vi "sortData.vi"(8 "error in (no error)":errorcluster, 9 "data":T1(array[cluster])=[[{"time"=0.0, "Channel"=refnum, "data"=0.8}, {"time"=29.998, "Channel"=refnum, "data"=0.0}], [{"time"=0.0, "Channel"=refnum, "data"=0.74}, {"time"=29.998, "Channel"=refnum, "data"=0.0}], [{"time"=29.998, "Channel"=refnum, "data"=0.8}, {"time"=33.5, "Channel"=refnum, "data"=0.0}]], 10 "times":dbl[](array[numeric]), 11 "ScriptEventList in":refnum<class "ScriptEventList.lvclass">) -> (0 "error out":errorcluster, 2 "data out":T1(array[cluster]), 3 "ScriptEventList out":refnum<class "ScriptEventList.lvclass">)   [LabVIEW 2009, in "Tools.lvlib" / "Scripting.lvlib" / "ScriptEventList.lvclass"]
uses:
  ScriptEventList.lvclass
  DatabaseHelpers/Database Objects/Channel/Channel.lvclass
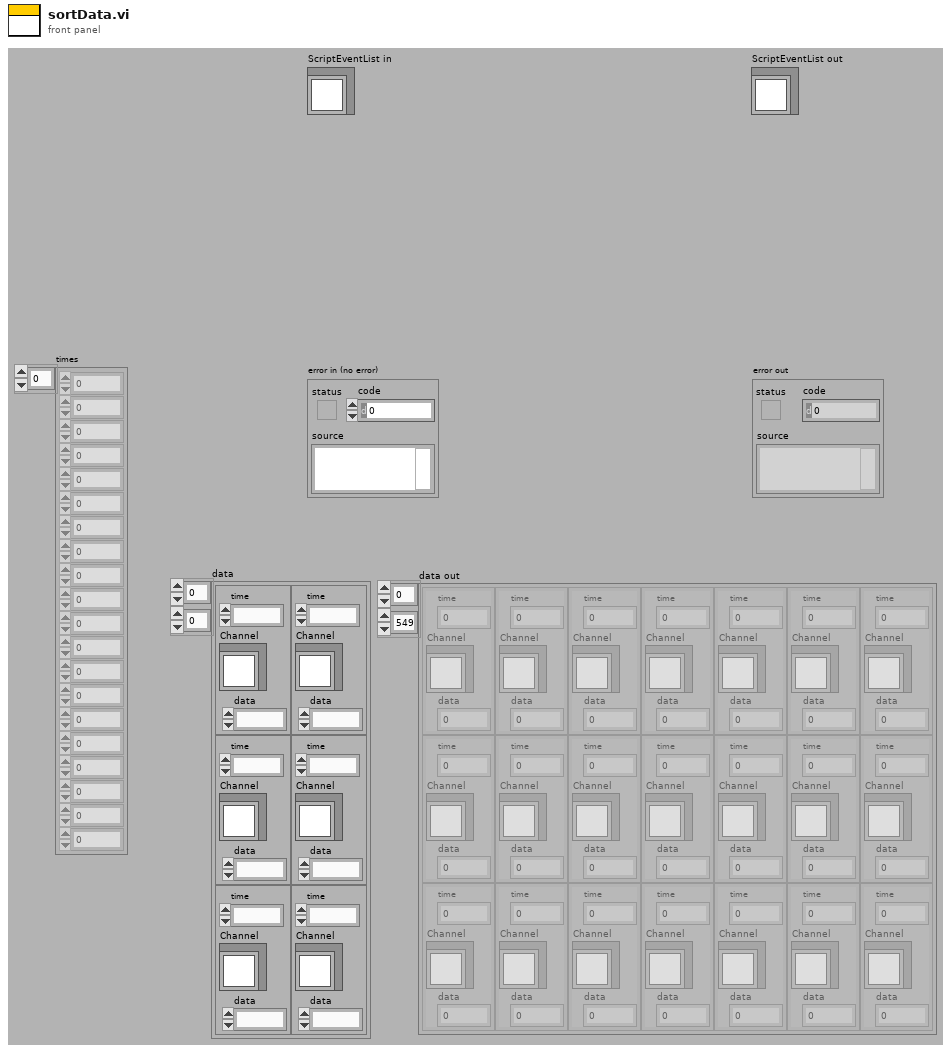
[diagram p1: front panel]
types:
  T1 = cluster{"time":dbl, "Channel":refnum<class "Channel.lvclass">, "data":dbl}[][]
  T2 = cluster{"time":dbl, "Channel":refnum<class "Channel.lvclass">, "data":dbl}[]
  T3 = cluster{"time":dbl, "Channel":refnum<class "Channel.lvclass">, "data":dbl}
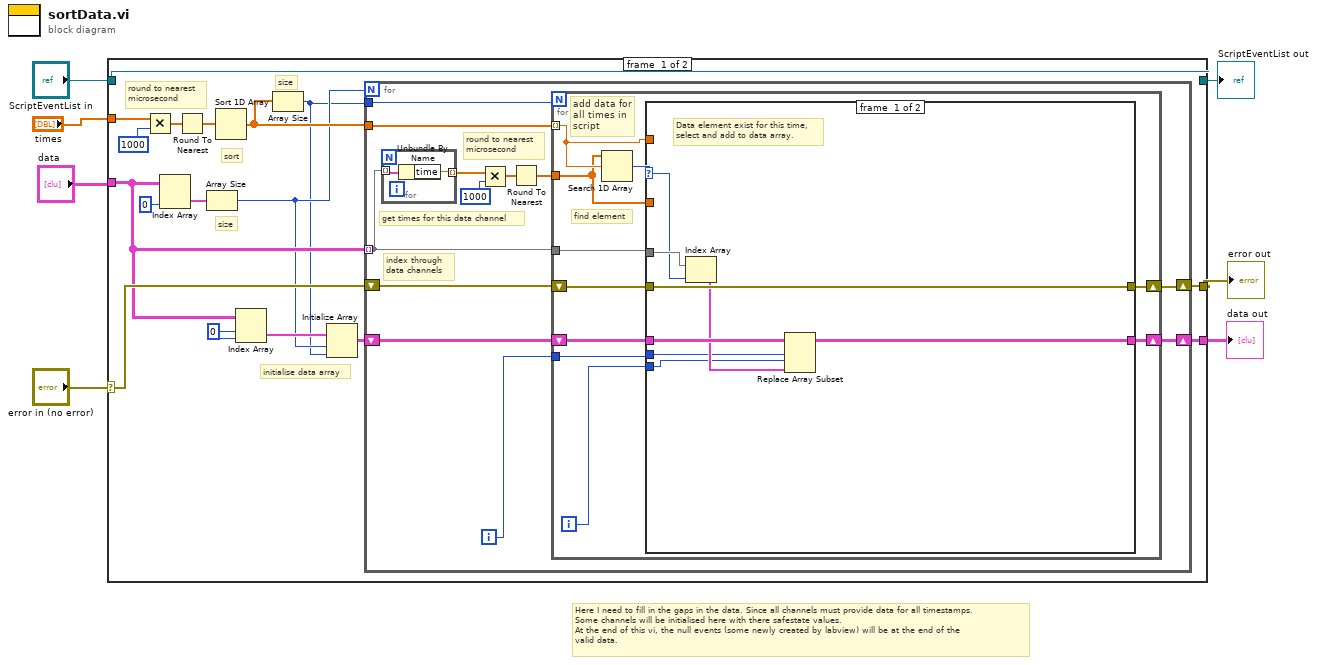
[diagram p0: block diagram]
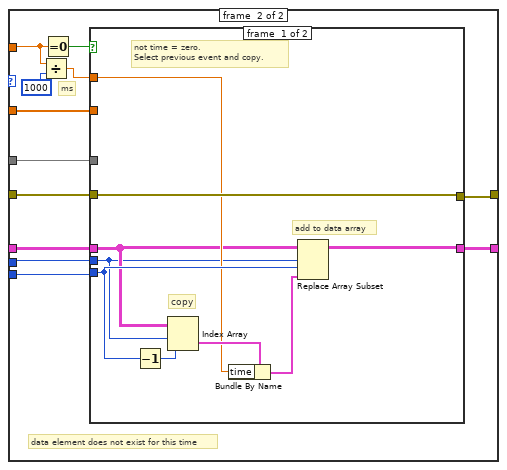
[diagram p2: hidden frame]
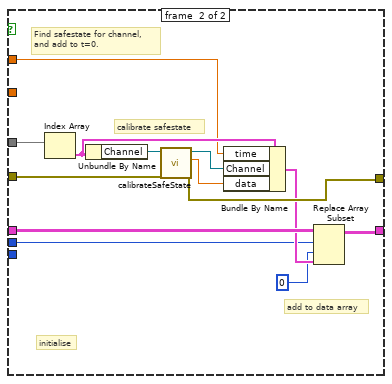
[diagram p3: hidden frame]
diagram:
  # "Here I need to fill in the gaps in the data. Since all channels must provide data for all timestamps.\nSome channels will be initialised here with there safestate values. \nAt the end of this vi, the null events (some newly created by labview) will be at the end of the \nvalid data."
  n1 = case shown="No Error" "error in (no error)" {
    selector: "error in (no error)" -> [w24 w92]
    tunnel: [w22 w92] -> w6
    tunnel: [w23 w91] -> w4
    tunnel: "ScriptEventList in" -> [w23 w91]
    tunnel: "times" -> [w11 _]
    tunnel: "data" -> [w20 _]
    tunnel: [w12 _] -> w1
    frame #0 {
      w18 = 0
      # "size"
      # "sort"
      # "round to nearest\nmicrosecond"
      # "initialise data array"
      # "size"
      n2 = Multiply(x=w11, y=1000) -> (x*y=w9:dbl[])
      n3 = Index Array(array=w20, index (col)=0) -> (element=w16:T2)  [unwired: 1 in]
      n4 = Round To Nearest(number=w9) -> (nearest integer value=w8:dbl[])
      n5 = Array Size(array=w16) -> (size(s)=w15:i32)
      n6 = Sort 1D Array(array=w8) -> (sorted array=w17:dbl[])
      n7 = Index Array(array=w20, index (row)=w18, index (col)=w18) -> (element=w19:T3)
      n8 = Array Size(array=w17) -> (size(s)=w14:i32)
      n9 = Initialize Array(w19, w15, w14) -> (w13:T1)
      n10 = for {
        N: w15 -> [_]
        tunnel: w17 -> [w34]
        shift-right: [w36] -> w22
        shift-left: w24 -> [w35]
        tunnel: w20 -> [w29] mode=indexing
        tunnel: w14 -> [w33]
        shift-right: [w30] -> w12
        shift-left: w13 -> [w32]
        i -> [w31]
        # "index through\ndata channels"
        # "get times for this data channel"
        # "round to nearest\nmicrosecond"
        n11 = for {
          tunnel: w29 -> [w37] mode=indexing
          tunnel: [w38] -> w26 mode=indexing
          n12 = Unbundle By Name(w37) -> ("time"=w38:dbl)
        }
        n13 = Multiply(x=w26, y=1000) -> (x*y=w28:dbl[])
        n14 = Round To Nearest(number=w28) -> (nearest integer value=w25:dbl[])
        n15 = for {
          N: w33 -> [_]
          shift-right: [w46] -> w36
          shift-left: w35 -> [w47]
          tunnel: w34 -> [w44] mode=indexing
          shift-right: [w40] -> w30
          shift-left: w32 -> [w43]
          tunnel: w31 -> [w42]
          tunnel: w25 -> [w39]
          tunnel: w29 -> [w45]
          i -> [w41]
          # "add data for \nall times in\nscript"
          # "find element"
          n16 = Search 1D Array(1D array=w39, element=w44) -> (index of element=w48:i32)  [unwired: 1 in]
          n17 = case shown="-1" w48 {
            selector: w48 -> [w50 _]
            tunnel: w44 -> [_ w59]
            tunnel: w39 -> [_ w67]
            tunnel: w45 -> [w53 w66]
            tunnel: w47 -> [w56 w65]
            tunnel: [w56 w64] -> w46
            tunnel: w41 -> [w49 w63]
            tunnel: w43 -> [w55 w62]
            tunnel: w42 -> [w51 w61]
            tunnel: [w54 w60] -> w40
            frame #0 {
              # "Data element exist for this time,\nselect and add to data array."
              n18 = Index Array(array=w53, index=w50) -> (element=w52:T3)
              n19 = Replace Array Subset(array=w55, new element=w52, index (row)=w51, index (col)=w49) -> (w54:T1)
            }
            frame #1 {
              # "ms"
              # "data element does not exist for this time"
              n20 = Divide(x=w59, y=1000) -> (x/y=w58:dbl)
              n21 = Equal To 0?(x=w59) -> (x = 0?=w68:bool)
              n22 = case shown="False" w68 {
                tunnel: w58 -> [w73 w87]
                tunnel: w67 -> [_ _]
                tunnel: w66 -> [_ w78]
                tunnel: w65 -> [w77 w89]
                tunnel: [w77 w85] -> w64
                tunnel: w63 -> [w75 _]
                tunnel: w62 -> [w71 w83]
                tunnel: w61 -> [w69 w79]
                tunnel: [w76 w81] -> w60
                frame #0 {
                  # "add to data array"
                  # "copy"
                  # "not time = zero.\nSelect previous event and copy."
                  n23 = Decrement(x=w75) -> (x-1=w70:i32)
                  n24 = Index Array(array=w71, index (row)=w69, index (col)=w70) -> (element=w74:T3)
                  n25 = Bundle By Name(cluster=w74, "time"=w73) -> (w72:T3)
                  n26 = Replace Array Subset(array=w71, new element=w72, index (row)=w69, index (col)=w75) -> (w76:T1)
                }
                frame #1 {
                  # "add to data array"
                  # "calibrate safestate"
                  # "Find safestate for channel,\nand add to t=0."
                  # "initialise"
                  n27 = Index Array(array=w78) -> (element=w88:T3)  [unwired: 1 in]
                  n28 = Unbundle By Name(w88) -> ("Channel"=w90:refnum<class "Channel.lvclass">)
                  n29 = call "calibrateSafeState.vi"("error in (no error)"=w89, "Channel in"=w90) -> ("error out"=w85:errorcluster, "calibratedValue"=w84:dbl, "Channel out"=w86:refnum<class "Channel.lvclass">)  [unwired: 7 in]
                  n30 = Bundle By Name(cluster=w88, "time"=w87, "Channel"=w86, "data"=w84) -> (w82:T3)
                  n31 = Replace Array Subset(array=w83, new element=w82, index (row)=w79, index (col)=0) -> (w81:T1)
                }
              }
            }
          }
        }
      }
    }
    frame #1 {
    }
  }
  "error out" <- w6
  "ScriptEventList out" <- w4
  "data out" <- w1
